vi "LED Color to RGB Percentages.vi"(10 "LED Color":u32(colorbox)) -> (1 "Blue %":u8, 2 "Green %":u8, 3 "Red %":u8)   [LabVIEW 2022 SP3, in "Logitech Devices.lvlib"]
uses:
  Logitech Devices.lvlib
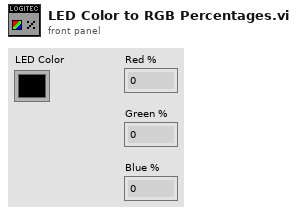
[diagram p1: front panel]
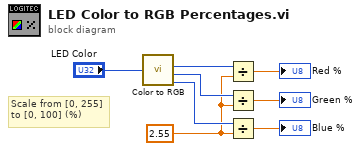
[diagram p0: block diagram]
diagram:
  w5 = 2.55 ("y")
  # "Scale from [0, 255]\nto [0, 100] (%)"
  n1 = call <vilib>:"Color to RGB.vi"("Color"="LED Color") -> ("R"=w8:u8, "G"=w7:u8, "B"=w6:u8)  [unwired: 1 out]
  n2 = Divide(x=w8, y=w5) -> (x/y=→"Red %":dbl)
  n3 = Divide(x=w7, y=w5) -> (x/y=→"Green %":dbl)
  n4 = Divide(x=w6, y=w5) -> (x/y=→"Blue %":dbl)
